vi "Exercise 3-5 Determine Warnings .vi"() -> ()   [LabVIEW 2014]
panel:
  in  "Current temp 2":dbl
  out "Boolean":bool
  out "String":string
  in  "minimum temp":dbl
  in  "max temp":dbl
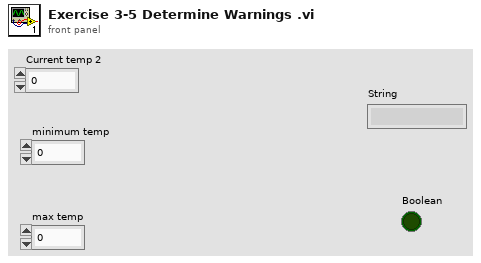
[diagram p1: front panel]
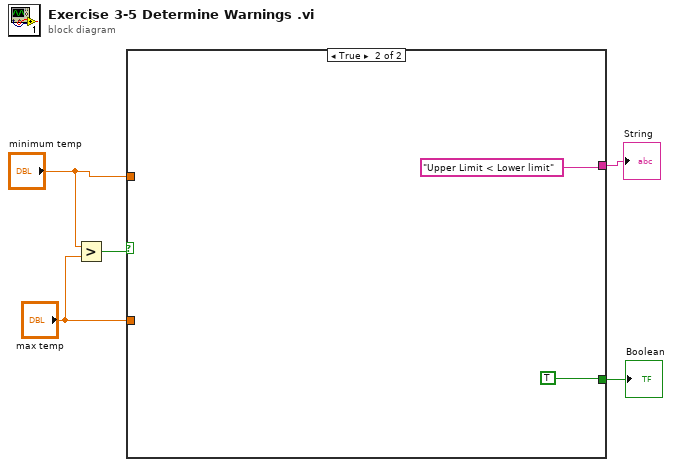
[diagram p0: block diagram]
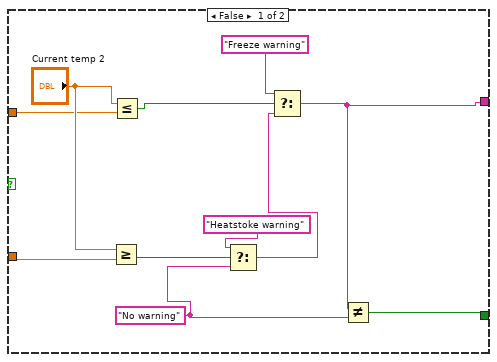
[diagram p2: hidden frame]
diagram:
  n1 = Greater?(x="minimum temp", y="max temp") -> (0:w3:bool)
  n2 = case shown="True" w3 {
    tunnel: [w8 "Upper Limit < Lower limit"] -> w5
    tunnel: [w9 TRUE] -> w4
    tunnel: "minimum temp" -> [w7 _]
    tunnel: "max temp" -> [w6 _]
    frame False {
      w11 = "No warning"
      n3 = Greater Or Equal?(x="Current temp 2", y=w6) -> (x >= y?=w16:bool)
      n4 = Less Or Equal?(x="Current temp 2", y=w7) -> (x <= y?=w15:bool)
      n5 = Select(t="Heatstoke warning", s=w16, f=w11) -> (s? t:f=w12:string)
      n6 = Select(t="Freeze warning", s=w15, f=w12) -> (s? t:f=w8:string)
      n7 = Not Equal?(x=w8, y=w11) -> (x != y?=w9:bool)
    }
    frame True {
    }
  }
  "String" <- w5
  "Boolean" <- w4
